vi "Gear Delivery Test.vi"   [LabVIEW 2016]
uses:
  <vilib>/Rock Robotics/WPI/Solenoid/WPI_SolenoidValue.ctl
  Global Variables/Refnum Names.vi
  <vilib>/Rock Robotics/WPI/Utilities/WPI_GetSetVariantRefNum.vi
  <vilib>/Rock Robotics/WPI/Solenoid/WPI_SolenoidSetEnum.vi
types:
  T1 = typedef "WPI_SolenoidDevRef.ctl" = cluster{"DevStatus":errorcluster, "Pneumatics Control Module":u8, "Forward Solenoid Channel":T2, "Reverse Solenoid Channel":T2}
  T2 = typedef "WPI_SolenoidChannel.ctl" = enum8{"Solenoid 0", "Solenoid 1", "Solenoid 2", "Solenoid 3", "Solenoid 4", "Solenoid 5", "Solenoid 6", "Solenoid 7", "Invalid"}
  T3 = typedef "WPI_JoystickDevRef.ctl" = cluster{"Device":T4}
  T4 = typedef "WPI_JoystickDeviceEnum.ctl" = enum16{"USB 0", "USB 1", "USB 2", "USB 3", "USB 4", "USB 5"}
  T5 = typedef "WPI_SolenoidValue.ctl" = enum16{"Off", "On", "Forward", "Reverse"}
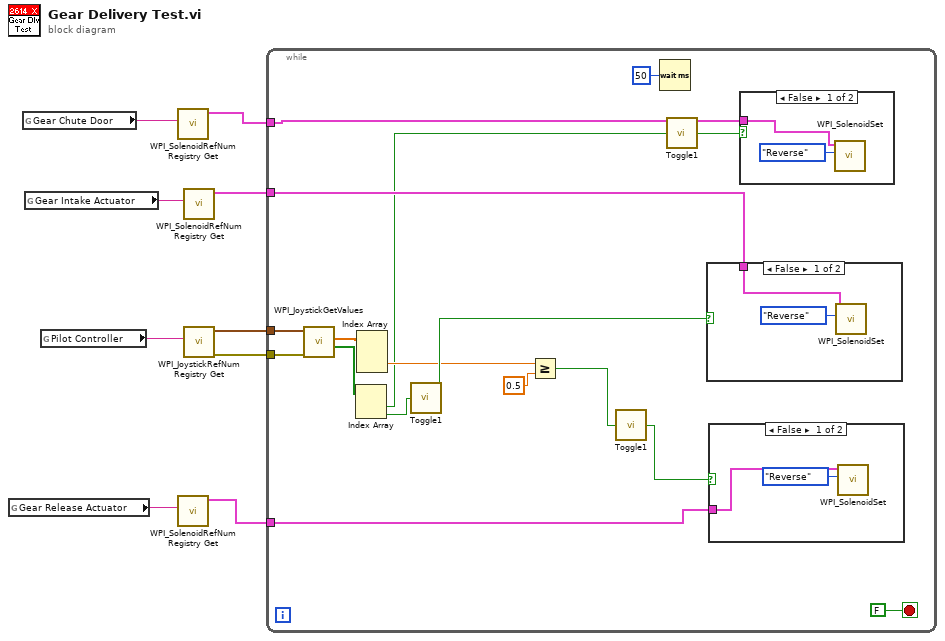
[diagram p0: block diagram]
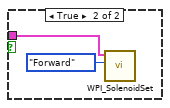
[diagram p2: hidden frame]
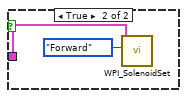
[diagram p3: hidden frame]
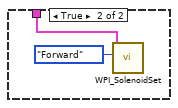
[diagram p4: hidden frame]
diagram:
  n1 = global read "Refnum Names.vi" "Gear Release Actuator"() -> (w9:string)
  n2 = global read "Refnum Names.vi" "Gear Chute Door"() -> (w2:string)
  n3 = global read "Refnum Names.vi" "Gear Intake Actuator"() -> (w8:string)
  n4 = global read "Refnum Names.vi" "Pilot Controller"() -> (w7:string)
  n5 = call <vilib>:"WPI_SolenoidRefNum Registry Get.vi"("refnum name"=w2) -> ("SolenoidDevRef"=w1:T1)  [unwired: 9 in, 1 out]
  n6 = call <vilib>:"WPI_SolenoidRefNum Registry Get.vi"("refnum name"=w9) -> ("SolenoidDevRef"=w3:T1)  [unwired: 9 in, 1 out]
  n7 = call <vilib>:"WPI_SolenoidRefNum Registry Get.vi"("refnum name"=w8) -> ("SolenoidDevRef"=w4:T1)  [unwired: 9 in, 1 out]
  n8 = call <vilib>:"WPI_JoystickRefNum Registry Get.vi"("refnum name"=w7) -> ("error out"=w5:errorcluster, "JoystickDevRef"=w6:T3)  [unwired: 9 in]
  n9 = while {
    tunnel: w6 -> [w23]
    tunnel: w5 -> [w24]
    tunnel: w4 -> [w20]
    tunnel: w3 -> [w13]
    tunnel: w1 -> [w10]
    stop <- FALSE stop-if-true
    n10 = call <vilib>:"WPI_JoystickGetValues.vi"("error in (no error)"=w24, "JoystickDevRef"=w23) -> ("Buttons"=w21:bool[], "Axes"=w22:dbl[])  [unwired: 5 in, 3 out]
    n11 = Index Array(array=w21) -> (element #1=w11:bool, element #2=w18:bool)  [unwired: 2 in]
    n12 = Index Array(array=w22) -> (element #3=w16:dbl)  [unwired: 3 in, 2 out]
    n13 = call "Toggle1.vi"("Boolean"=w18) -> ("Driver Switch 2"=w19:bool)
    n14 = Greater Or Equal?(x=w16, y=0.5) -> (x >= y?=w17:bool)
    n15 = call "Toggle1.vi"("Boolean"=w17) -> ("Driver Switch 2"=w14:bool)
    n16 = Wait (ms)(milliseconds to wait=u32 50) -> ()  [unwired: 1 out]
    n17 = call "Toggle1.vi"("Boolean"=w11) -> ("Driver Switch 2"=w12:bool)
    n18 = case shown="False" w19 {
      tunnel: w20 -> [w35 w38]
      frame False {
        n19 = call-poly <vilib>:"WPI_SolenoidSet.vi"("Value"=WPI_SolenoidValue."Reverse", "SolenoidDevRef"=w35) -> ()  [unwired: 8 in, 2 out]
      }
      frame True {
        n20 = call-poly <vilib>:"WPI_SolenoidSet.vi"("Value"=WPI_SolenoidValue."Forward", "SolenoidDevRef"=w38) -> ()  [unwired: 8 in, 2 out]
      }
    }
    n21 = case shown="False" w14 {
      tunnel: w13 -> [w31 w34]
      frame False {
        n22 = call-poly <vilib>:"WPI_SolenoidSet.vi"("Value"=WPI_SolenoidValue."Reverse", "SolenoidDevRef"=w31) -> ()  [unwired: 8 in, 2 out]
      }
      frame True {
        n23 = call-poly <vilib>:"WPI_SolenoidSet.vi"("Value"=WPI_SolenoidValue."Forward", "SolenoidDevRef"=w34) -> ()  [unwired: 8 in, 2 out]
      }
    }
    n24 = case shown="False" w12 {
      tunnel: w10 -> [w27 w29]
      frame False {
        n25 = call-poly <vilib>:"WPI_SolenoidSet.vi"("Value"=WPI_SolenoidValue."Reverse", "SolenoidDevRef"=w27) -> ()  [unwired: 8 in, 2 out]
      }
      frame True {
        n26 = call-poly <vilib>:"WPI_SolenoidSet.vi"("Value"=WPI_SolenoidValue."Forward", "SolenoidDevRef"=w29) -> ()  [unwired: 8 in, 2 out]
      }
    }
  }
